vi "Read Limits File.vi"(0 "Limits File Path":path, 11 "error in (no error)":errorcluster) -> (4 "Limit Data":T1, 15 "error out":errorcluster)   [LabVIEW 2020]
doc: "Read Limits File reads the expected waveform from the Limits file location."
uses:
  Plot Data.ctl
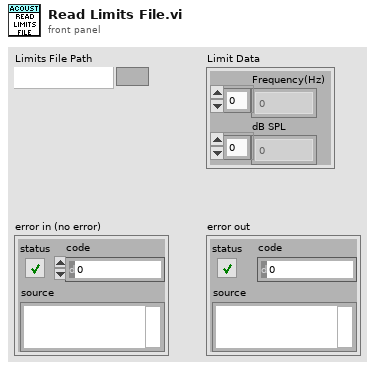
[diagram p1: front panel]
types:
  T1 = typedef "Plot Data.ctl" = cluster{"Frequency(Hz)":dbl[], "dB SPL":dbl[]}
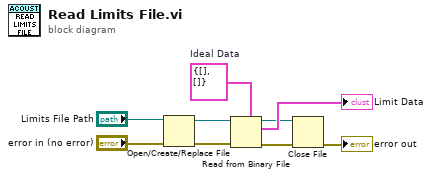
[diagram p0: block diagram]
diagram:
  w1 = T1 {"Frequency(Hz)"=[], "dB SPL"=[]}  # Ideal Data
  n1 = Open/Create/Replace File(file path (use dialog)="Limits File Path", error in="error in (no error)") -> (refnum out=w6:refnum<file>, error out=w5:errorcluster)  [unwired: 4 in, 1 out]
  n2 = Read from Binary File(5:w1, 8:w5, 11:w6) -> (0:w3:errorcluster, 2:→"Limit Data":T1, 3:w2:refnum<file>)  [unwired: 3 in, 1 out]
  n3 = Close File(refnum=w2, error in=w3) -> (error out=→"error out":errorcluster)  [unwired: 1 out]
